vi "~big config panel.vi"() -> ()   [LabVIEW 2017]
uses:
  Classes/Sequence/SequenceSubvis/TestStep-StepType.ctl
  Classes/Sequence/SequenceSubvis/RF Direction.ctl
  Classes/Sequence/SequenceSubvis/PolarizationSelect.ctl
  Classes/Sequence/SequenceSubvis/TestStepTypes.ctl
panel:
  out "TestSequence":T1[](array[typedef])
  in  "Cancel":bool
  in  "OK":bool
  in  "module 7":T5
  in  "module 6":T5
  in  "module 5":T5
  in  "module 4":T5
  in  "module 3":T5
  in  "module 2":T5
  in  "module 1":T5
  in  "module 0":T5
  # "Module 0"
  # "Module 1"
  # "Module 2"
  # "Module 3"
  # "Module 4"
  # "Module 5"
  # "Module 6"
  # "Module 7"
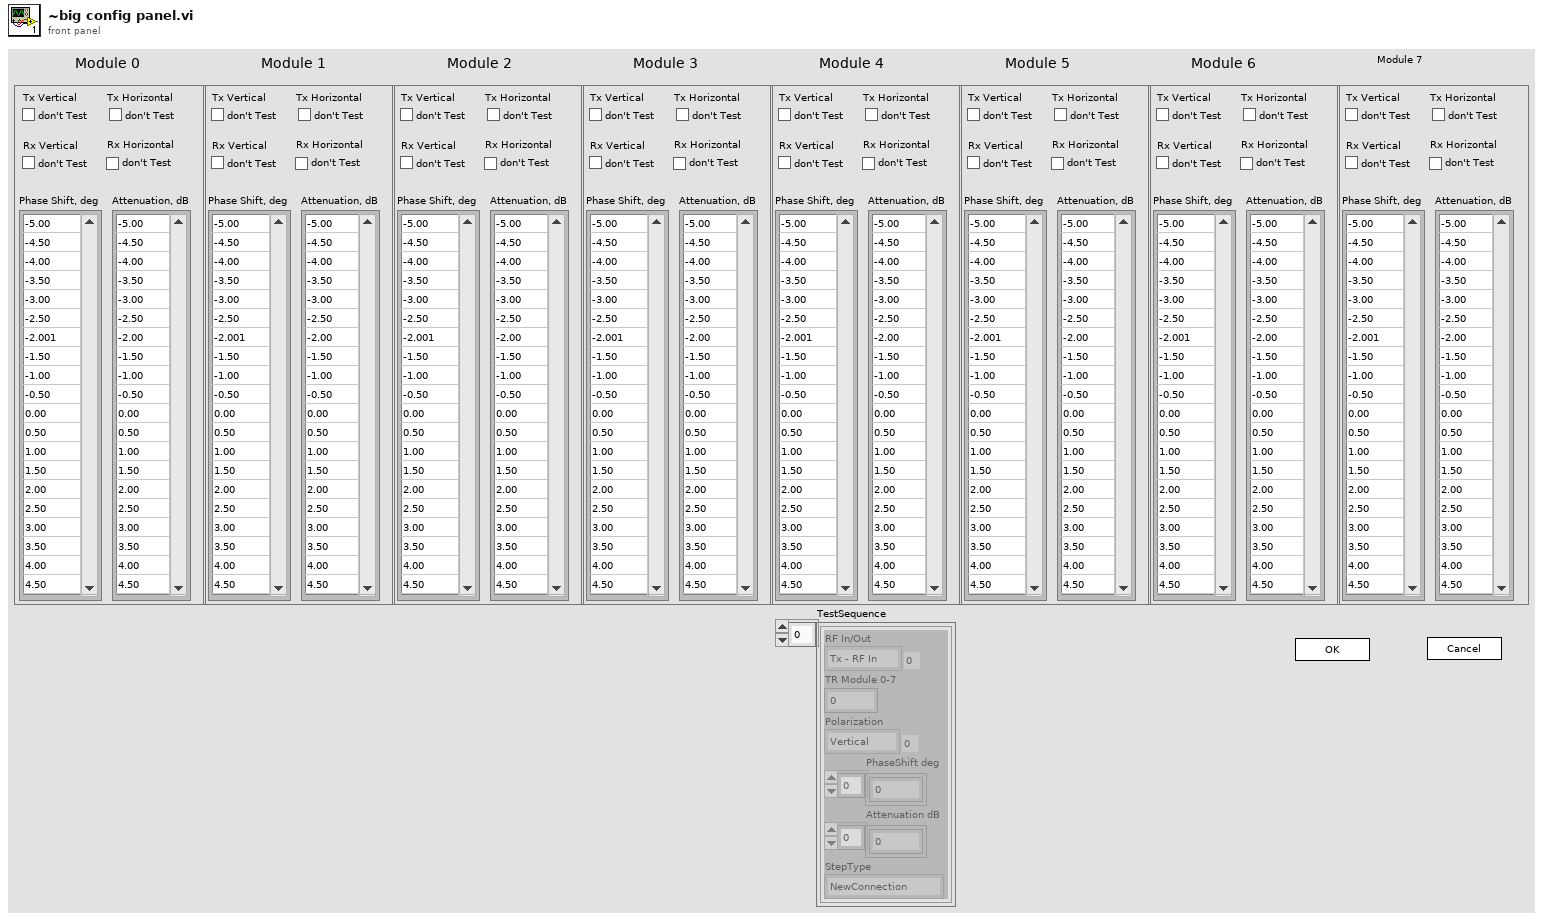
[diagram p1: front panel]
types:
  T1 = typedef "TestStep-StepType.ctl" = cluster{"RF In/Out":T2, "TR Module 0-7":i32, "Polarization":T3, "PhaseShift deg":dbl[], "Attenuation dB":dbl[], "StepType":T4}
  T2 = typedef "RF Direction.ctl" = enum16{"Tx - RF In", "Rx - RF Out"}
  T3 = typedef "PolarizationSelect.ctl" = enum16{"Vertical", "Horizontal"}
  T4 = typedef "TestStepTypes.ctl" = enum16{"NewConnection", "SweepTest", "Motion", "Finish"}
  T5 = cluster{"Tx Vertical":bool, "Tx Horizontal":bool, "Rx Vertical":bool, "Rx Horizontal":bool, "Attenuation, dB":i32[], "Phase Shift, deg":i32[]}
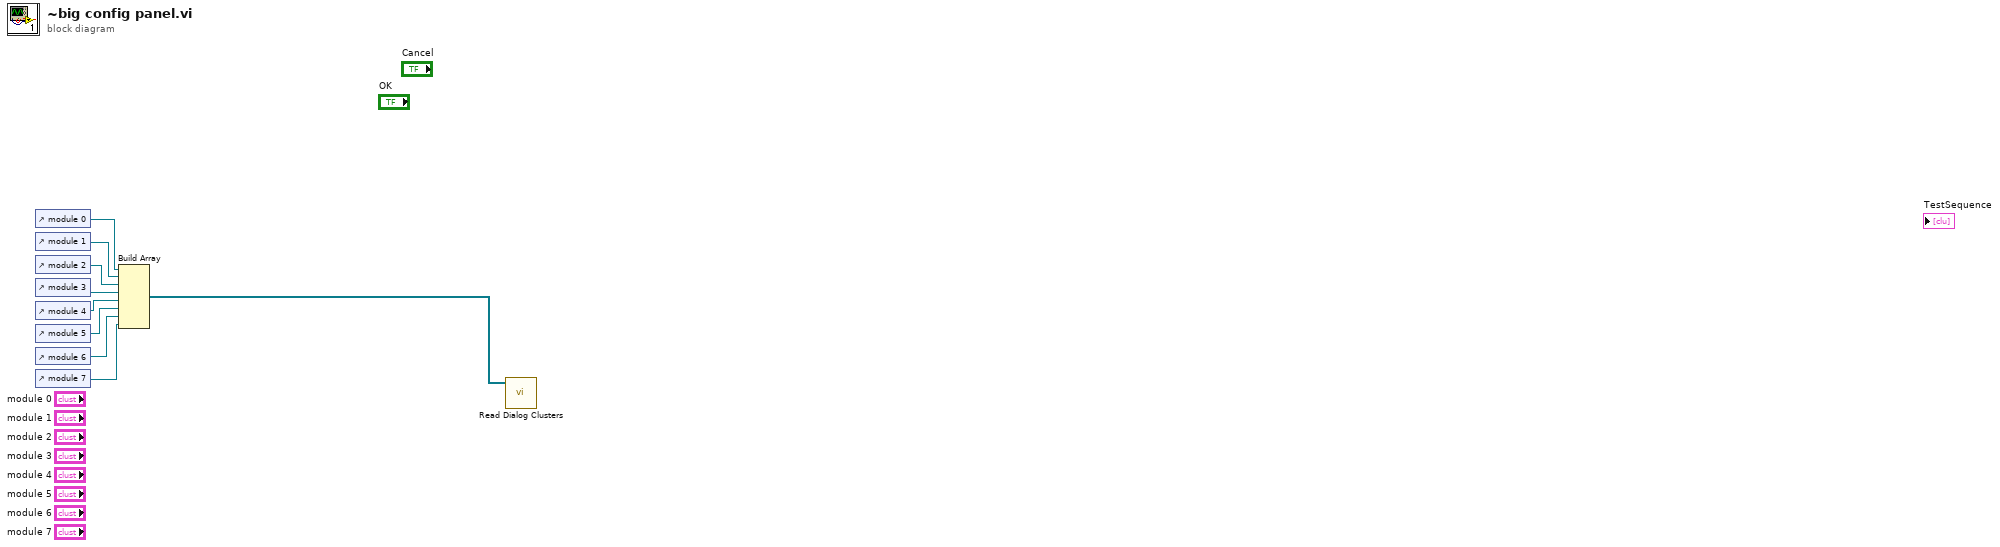
[diagram p0: block diagram]
diagram:
  n1 = control-ref of="module 0"() -> (w8:refnum<vi>)
  n2 = control-ref of="module 1"() -> (w7:refnum<vi>)
  n3 = control-ref of="module 2"() -> (w6:refnum<vi>)
  n4 = control-ref of="module 3"() -> (w5:refnum<vi>)
  n5 = control-ref of="module 4"() -> (w4:refnum<vi>)
  n6 = control-ref of="module 5"() -> (w3:refnum<vi>)
  n7 = control-ref of="module 6"() -> (w2:refnum<vi>)
  n8 = control-ref of="module 7"() -> (w1:refnum<vi>)
  n9 = Build Array(w8, w7, w6, w5, w4, w3, w2, w1) -> (w9:refnum<vi>[])
  n10 = call "Read Dialog Clusters.vi"("Module Cluster Refs"=w9) -> ()  [unwired: 10 in, 1 out]
